vi "subPolyCoeff.vi"(10 "theta":dbl, 11 "r":dbl) -> (3 "Coeff":dbl[](array[numeric]))   [LabVIEW 2011]
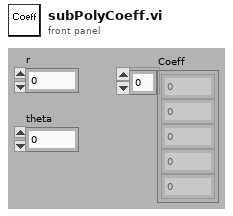
[diagram p1: front panel]
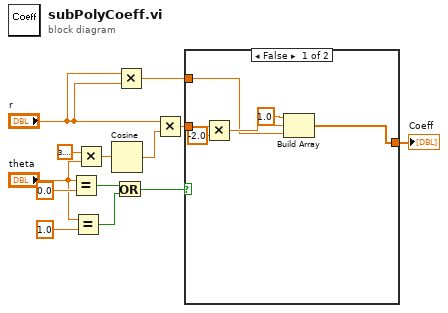
[diagram p0: block diagram]
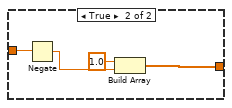
[diagram p2: hidden frame]
diagram:
  n1 = Equal?(x="theta", y=0.0) -> (x = y?=w11:bool)
  n2 = Equal?(x="theta", y=1.0) -> (x = y?=w10:bool)
  n3 = Multiply(x=3.141592653589793, y="theta") -> (x*y=w3:dbl)
  n4 = Cosine(x=w3) -> (cos(x)=w7:dbl)
  n5 = Or(x=w11, y=w10) -> (x .or. y?=w9:bool)
  n6 = Multiply(x="r", y="r") -> (x*y=w8:dbl)
  n7 = Multiply(x="r", y=w7) -> (x*y=w6:dbl)
  n8 = case shown="False" w9 {
    tunnel: w8 -> [w15 _]
    tunnel: w6 -> [w18 w22]
    tunnel: [w14 w20] -> w4
    frame False {
      n9 = Multiply(x=w18, y=-2.0) -> (x*y=w16:dbl)
      n10 = Build Array(1.0 ("element"), w16, w15) -> (w14:dbl[])
    }
    frame True {
      n11 = Negate(x=w22) -> (-x=w21:dbl)
      n12 = Build Array(1.0 ("element"), w21) -> (w20:dbl[])
    }
  }
  "Coeff" <- w4
